vi "方波子vi.vi"(10 "幅值":dbl) -> (2 "数组":dbl[](array[numeric]))   [LabVIEW 2018]
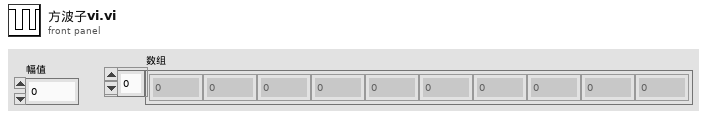
[diagram p1: front panel]
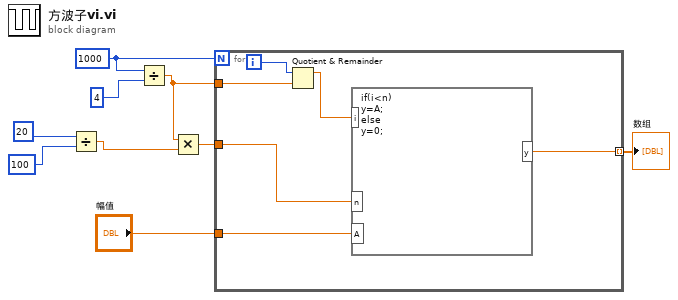
[diagram p0: block diagram]
diagram:
  w8 = 1000
  n1 = Divide(x=20, y=100) -> (x/y=w2:dbl)
  n2 = Divide(x=w8, y=4) -> (x/y=w3:dbl)
  n3 = Multiply(x=w3, y=w2) -> (x*y=w1:dbl)
  n4 = for {
    N: w8 -> [_]
    tunnel: w3 -> [w12]
    tunnel: "幅值" -> [w13]
    tunnel: [w11] -> w6 mode=indexing
    tunnel: w1 -> [w10]
    i -> [w15]
    n5 = Quotient & Remainder(x=w15, y=w12) -> (x-y*floor(x/y)=w14:dbl)  [unwired: 1 out]
    n6 = formula code="if(i<n)\ny=A;\nelse\ny=0;"("i"=w14, "A"=w13, "n"=w10) -> ("y"=w11:dbl)
  }
  "数组" <- w6
